vi "Pre Launch Init.vi"(11 "Analog Reader in":refnum<class "Analog Reader.lvclass">) -> (0 "error out":errorcluster, 3 "Analog Reader out":refnum<class "Analog Reader.lvclass">)   [LabVIEW 2024, in "DAQmx Actor.lvlib" / "Analog Reader.lvclass"]
doc: "<p>(<strong>Filename</strong>: <span class=\"dnl\">Actor Framework.lvlib:Actor.lvclass:Pre Launch Init.vi</span>)</p>\n<p>Defines behavior that occurs after the <a href=\"nihelplauncher://docs/csh?context=lvcore_lvcomm_af_launch_nested_actor\">Launch Nested Actor</a> method is invoked but before the actor's Actor Core method begins running.</p>\n<p>By default, this method does nothing. A descendant class may override it to define behavior.</p>"
uses:
  Analog Reader.lvclass
  DAQmx Actor/DAQmx Actor.lvclass
  Analog Reader.lvclass/Analog Reader.ctl
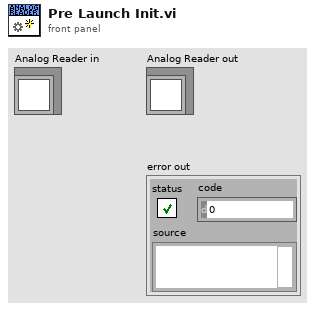
[diagram p1: front panel]
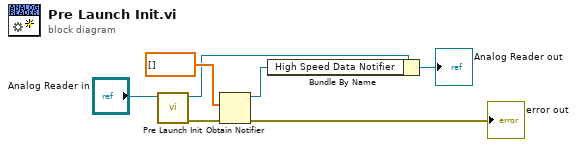
[diagram p0: block diagram]
diagram:
  n1 = call-parent "Pre Launch Init.vi"("DAQmx Actor in"="Analog Reader in") -> ("error out"=w6:errorcluster, "DAQmx Actor out"=w3:refnum<class "Analog Reader.lvclass">)  [unwired: 9 in]
  n2 = Obtain Notifier(notification data type=dbl[] [], error in (no error)=w6) -> (notifier out=w2:refnum<notifier>, error out=→"error out":errorcluster)  [unwired: 2 in, 1 out]
  n3 = Bundle By Name(cluster=w3, "High Speed Data Notifier"=w2) -> (→"Analog Reader out":refnum<class "Analog Reader.lvclass">)
